vi "BRig_dataMTrig_Audio_T_R.vi"() -> (2 "output_Audio_T_R":i32)   [LabVIEW 2014]
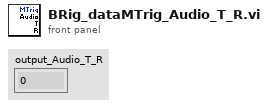
[diagram p1: front panel]
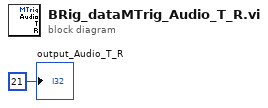
[diagram p0: block diagram]
diagram:
  "output_Audio_T_R" <- 21 ("output_iBlock")
